vi "Get envelope and Phase.vi"(8 "thickness":i32, 11 "signal":dbl[](array[numeric])) -> (0 "phase":dbl, 3 "envelope":dbl)   [LabVIEW 2017]
uses:
  <vilib>/Analysis/NI_AALPro.lvlib
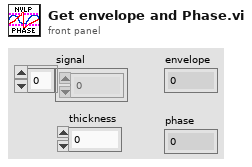
[diagram p1: front panel]
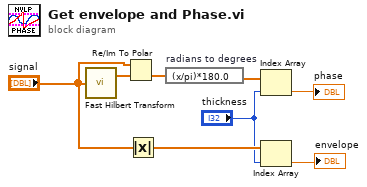
[diagram p0: block diagram]
diagram:
  n1 = call <vilib>:"Fast Hilbert Transform.vi"("X"="signal") -> ("Hilbert{X}"=w6:dbl[])  [unwired: 1 out]
  n2 = Re/Im To Polar(2:w6, 3:"signal") -> (0:w7:dbl[])  [unwired: 1 out]
  n3 = Absolute Value(x="signal") -> (abs(x)=w4:dbl[])
  n4 = expression code="(x/pi)*180.0" "radians to degrees"(w7) -> (w8:dbl[])
  n5 = Index Array(array=w8, index="thickness") -> (element=→"phase":dbl)
  n6 = Index Array(array=w4, index="thickness") -> (element=→"envelope":dbl)
